vi "Facade.vi"(0 "Data In":T5, 2 "Display State In":T3, 3 "Container State":T4) -> (6 "Data Out":T5, 7 "Display State Out":T3, 8 "Action":T2)   [LabVIEW 2019, in "XControllerSettings.xctl"]
uses:
  XControllerSettings.xctl
  Data.ctl
  <vilib>/_xctls/Container State.ctl
  State.ctl
  <vilib>/_xctls/Action.ctl
  <vilib>/_xctls/XControlSupport.lvlib
panel:
  in  "ControllerSettings":T1
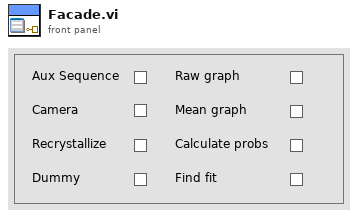
[diagram p1: front panel]
types:
  T1 = cluster{"Aux Sequence":bool, "Camera":bool, "Recrystallize":bool, "Raw graph":bool, "Mean graph":bool, "Calculate probs":bool, "Find fit":bool, "Dummy":bool}
  T2 = typedef "XControlSupport.lvlib/Action.ctl" = cluster{"Data Changed?":bool, "State Changed?":bool, "Action Name":string}
  T3 = typedef "XControllerSettings.xctl/State.ctl" = cluster{"Aux Sequence":bool, "Camera":bool, "Recrystallize":bool, "Raw graph":bool, "Mean graph":bool, "Calculate probs":bool, "Find fit":bool, "Dummy":bool}
  T4 = typedef "XControlSupport.lvlib/Container State.ctl" = cluster{"Indicator?":bool, "Run Mode?":bool, " Refnum":refnum<vi>}
  T5 = typedef "XControllerSettings.xctl/Data.ctl" = cluster{"Aux Sequence":bool, "Camera":bool, "Recrystallize":bool, "Raw graph":bool, "Mean graph":bool, "Calculate probs":bool, "Find fit":bool, "Dummy":bool}
  T6 = enum8{"Enabled", "Disabled", "Disabled and Grayed Out"}
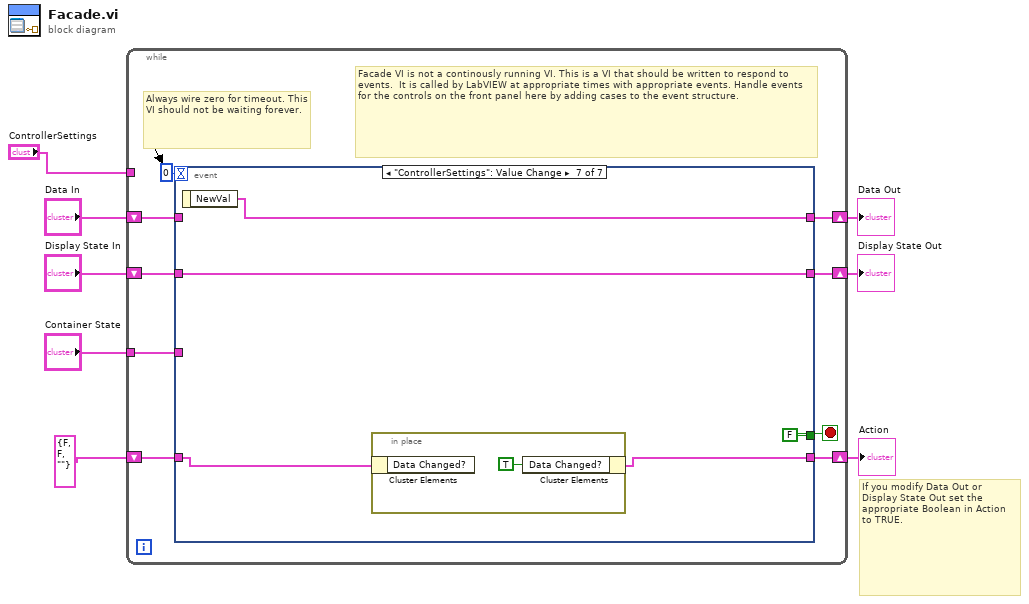
[diagram p0: block diagram]
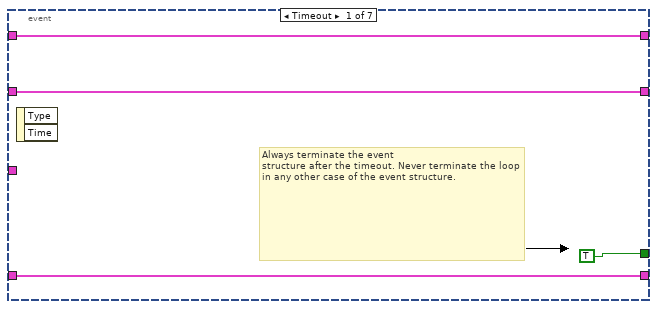
[diagram p2: hidden frame]
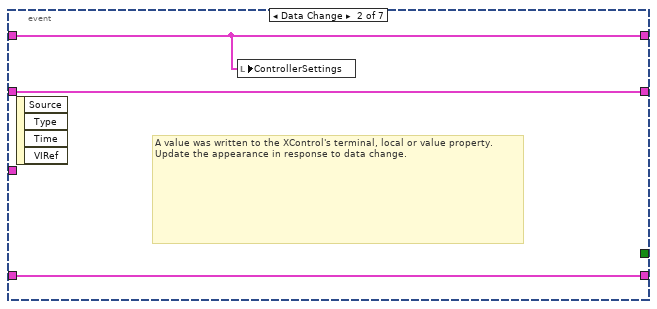
[diagram p3: hidden frame]
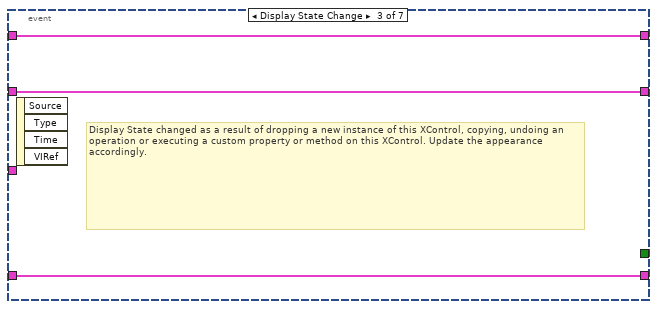
[diagram p4: hidden frame]
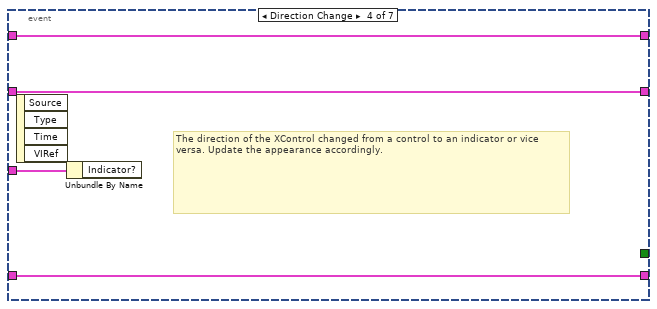
[diagram p5: hidden frame]
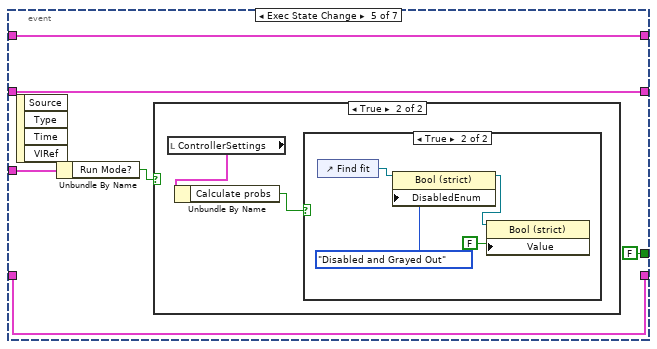
[diagram p6: hidden frame]
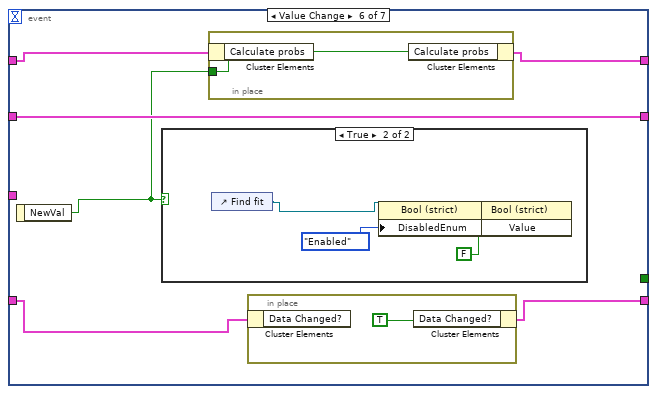
[diagram p9: hidden frame]
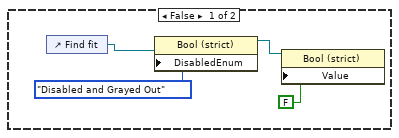
[diagram p10: hidden frame]
diagram:
  # "If you modify Data Out or\nDisplay State Out set the\nappropriate Boolean in Action\nto TRUE."
  n1 = while {
    shift-right: [w16] -> w5
    shift-left: "Display State In" -> [w17]
    tunnel: "Container State" -> [w13]
    shift-right: [w11] -> w8
    shift-left: "Data In" -> [w12]
    shift-right: [w9] -> w3
    shift-left: T2 {"Data Changed?"=FALSE, "State Changed?"=FALSE, "Action Name"=""} ("Action") -> [w10]
    tunnel: "ControllerSettings" -> [_]
    stop <- w15 stop-if-true
    # "Facade VI is not a continously running VI. This is a VI that should be written to respond to events.  It is called by LabVIEW at appropriate times with appropriate events. Handle events for the controls on the front panel here by adding cases to the event structure."
    # "Always wire zero for timeout. This\nVI should not be waiting forever."
    n2 = event shown="[6] \"ControllerSettings\": Value Change" {
      selector: _ -> [_ _ _ _ _ _ _]
      dyn-events: _ -> [_ _ _ _ _ _ _]
      timeout: 0 -> [_ _ _ _ _ _ _]
      tunnel: w17 -> [w19 w24 w27 w30 w36 w49 w64]
      tunnel: [w19 w24 w27 w30 w36 w49 w64] -> w16
      tunnel: [TRUE _ _ _ FALSE _ FALSE] -> w15
      tunnel: w13 -> [_ _ _ w31 w37 _ _]
      tunnel: w12 -> [w18 w22 w26 w29 w35 w46 _]
      tunnel: [w18 w22 w26 w29 w35 w44 w63] -> w11
      tunnel: [w20 w23 w25 w28 w34 w47 w60] -> w9
      tunnel: w10 -> [w20 w23 w25 w28 w34 w48 w61]
      event Timeout {
        # "Always terminate the event\nstructure after the timeout. Never terminate the loop in any other case of the event structure."
        n3 = event-data() -> ()  [unwired: 1 in, 2 out]
      }
      event Data Change {
        # "A value was written to the XControl's terminal, local or value property.\nUpdate the appearance in response to data change."
        n4 = event-data() -> ()  [unwired: 1 in, 4 out]
        n5 = local write "ControllerSettings"(w22) -> ()
      }
      event Display State Change {
        # "Display State changed as a result of dropping a new instance of this XControl, copying, undoing an operation or executing a custom property or method on this XControl. Update the appearance accordingly."
        n6 = event-data() -> ()  [unwired: 1 in, 4 out]
      }
      event Direction Change {
        # "The direction of the XControl changed from a control to an indicator or vice versa. Update the appearance accordingly."
        n7 = event-data() -> ()  [unwired: 1 in, 4 out]
        n8 = Unbundle By Name(w31) -> ()  [unwired: 1 out]
      }
      event Exec State Change {
        n9 = event-data() -> ()  [unwired: 1 in, 4 out]
        n10 = Unbundle By Name(w37) -> ("Run Mode?"=w33:bool)
        n11 = case shown="True" w33 {
          frame False {
          }
          frame True {
            n12 = local read "ControllerSettings"() -> (w39:T1)
            n13 = Unbundle By Name(w39) -> ("Calculate probs"=w38:bool)
            n14 = case shown="True" w38 {
              frame False {
              }
              frame True {
                n15 = control-ref of="Find fit"() -> (w43:refnum<vi>)
                n16 = property class="Bool (strict)"(reference=w43, "DisabledEnum"=T6."Disabled and Grayed Out" ("Disabled")) -> (reference out=w41:refnum<vi>)  [unwired: 1 in, 1 out]
                n17 = property class="Bool (strict)"(reference=w41, "Value"=FALSE) -> ()  [unwired: 1 in, 2 out]
              }
            }
          }
        }
      }
      event "ControllerSettings.Calculate probs": Value Change {
        n18 = event-data() -> ("NewVal"=w45:bool)  [unwired: 1 in]
        n19 = case shown="True" w45 {
          frame False {
            n20 = control-ref of="Find fit"() -> (w52:refnum<vi>)
            n21 = property class="Bool (strict)"(reference=w52, "DisabledEnum"=T6."Disabled and Grayed Out" ("Disabled")) -> (reference out=w54:refnum<vi>)  [unwired: 1 in, 1 out]
            n22 = property class="Bool (strict)"(reference=w54, "Value"=FALSE) -> ()  [unwired: 1 in, 2 out]
          }
          frame True {
            n23 = control-ref of="Find fit"() -> (w56:refnum<vi>)
            n24 = property class="Bool (strict)"(reference=w56, "DisabledEnum"=T6."Enabled" ("Disabled")) -> (reference out=w58:refnum<vi>)  [unwired: 1 in, 1 out]
            n25 = property class="Bool (strict)"(reference=w58, "Value"=FALSE) -> ()  [unwired: 1 in, 2 out]
          }
        }
        n26 = in-place {
          in-place-border: w45 -> [w50]
          n27 = in-place-cluster #1(w46) -> ()  [unwired: 1 out]
          n28 = in-place-cluster #1("Calculate probs"=w50) -> (w44:T5)
        }
        n29 = in-place {
          n30 = in-place-cluster #2(w48) -> ()  [unwired: 1 out]
          n31 = in-place-cluster #2("Data Changed?"=TRUE) -> (w47:T2)
        }
      }
      event "ControllerSettings": Value Change {
        n32 = event-data() -> ("NewVal"=w63:T1)  [unwired: 1 in]
        n33 = in-place {
          n34 = in-place-cluster #3(w61) -> ()  [unwired: 1 out]
          n35 = in-place-cluster #3("Data Changed?"=TRUE) -> (w60:T2)
        }
      }
    }
  }
  "Display State Out" <- w5
  "Data Out" <- w8
  "Action" <- w3
